vi "Get 24 Channels of Adam VDC.vi"() -> (0 "error out":errorcluster, 1 "TC Data":dbl[](array[numeric]), 2 "Analog Data Out":dbl[](array[numeric]))   [LabVIEW 2014, in "UI Core.lvlib"]
uses:
  VIs/UI Core.lvlib
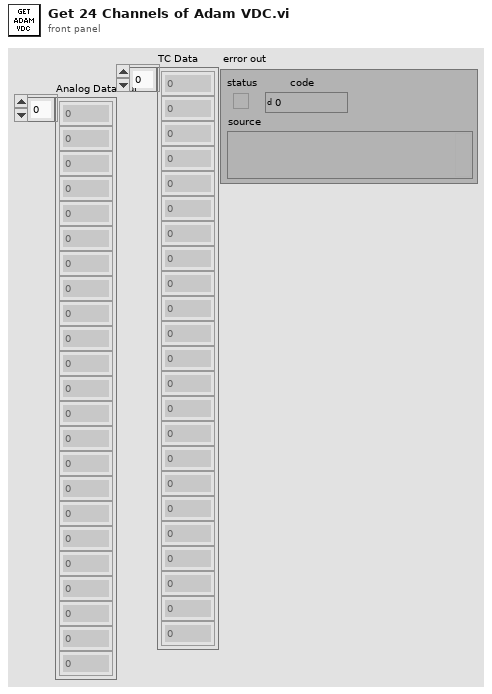
[diagram p1: front panel]
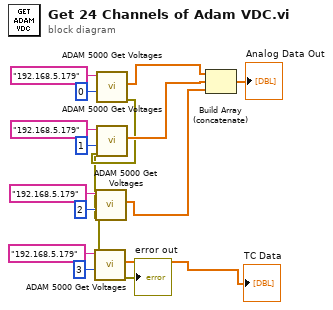
[diagram p0: block diagram]
diagram:
  n1 = call "ADAM 5000 Get Voltages.vi"("Bd # (0=first bd)"=u16 0, "Remote IP Address 2"="192.168.5.179") -> ("error out"=w4:errorcluster, "Data"=w15:dbl[])  [unwired: 7 in, 1 out]
  n2 = call "ADAM 5000 Get Voltages.vi"("error in (no error)"=w4, "Bd # (0=first bd)"=u16 1, "Remote IP Address 2"="192.168.5.179") -> ("error out"=w3:errorcluster, "Data"=w10:dbl[])  [unwired: 6 in, 1 out]
  n3 = call "ADAM 5000 Get Voltages.vi"("error in (no error)"=w3, "Bd # (0=first bd)"=u16 2, "Remote IP Address 2"="192.168.5.179") -> ("error out"=w2:errorcluster, "Data"=w9:dbl[])  [unwired: 6 in, 1 out]
  n4 = call "ADAM 5000 Get Voltages.vi"("error in (no error)"=w2, "Bd # (0=first bd)"=u16 3, "Remote IP Address 2"="192.168.5.179") -> ("error out"=→"error out":errorcluster, "Data"=→"TC Data":dbl[])  [unwired: 6 in, 1 out]
  n5 = Build Array (concatenate)(w15, w10, w9) -> (→"Analog Data Out":dbl[])
